vi "Recieve Status.vi"(8 "error in (no error)":errorcluster, 9 "Status offset":u64, 10 "Read config instead":bool, 11 "RP Communicator in":refnum<class "RP Communicator.lvclass">) -> (0 "error out":errorcluster, 1 "Status response":u32=1 format="0x%x (%d)", 3 "RP Communicator out":refnum<class "RP Communicator.lvclass">)   [LabVIEW 2016, in "RP Communicator.lvclass"]
uses:
  RP Communicator.lvclass
  RP Communicator.lvclass/RP Communicator.ctl
  Read Timeout.vi
  RP Read Status TCP.vi
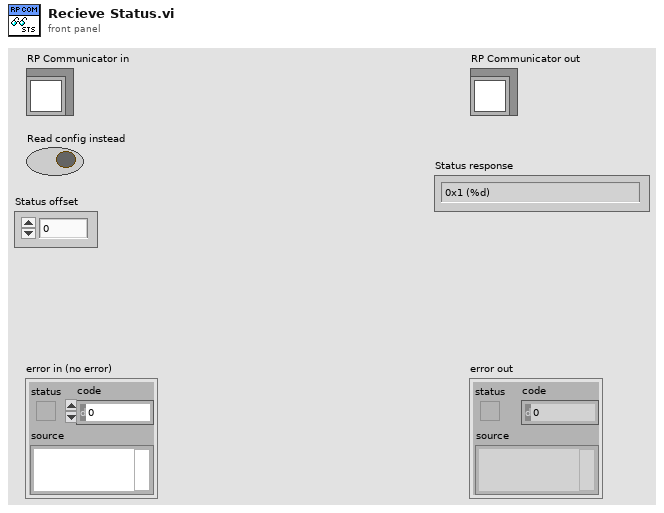
[diagram p1: front panel]
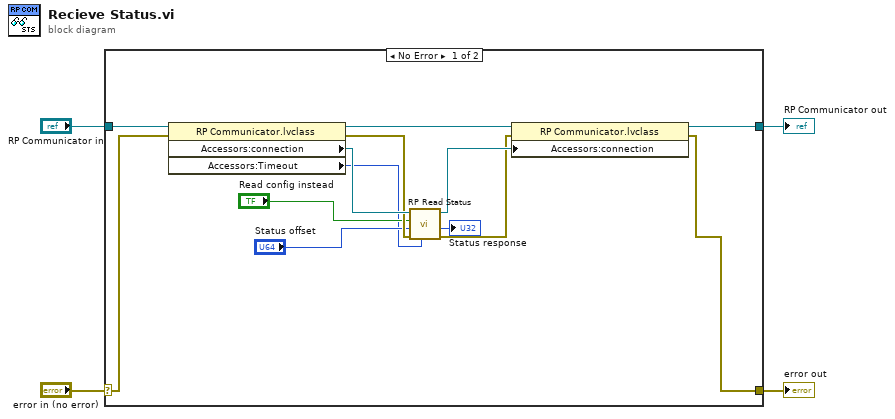
[diagram p0: block diagram]
diagram:
  n1 = case shown="No Error" "error in (no error)" {
    selector: "error in (no error)" -> [w9 w19]
    tunnel: [w11 w19] -> w3
    tunnel: [w14 w18] -> w1
    tunnel: "RP Communicator in" -> [w17 w18]
    frame No Error {
      n2 = property class="RP Communicator.lvclass"(reference=w17, error in=w9) -> (reference out=w16:refnum<class "RP Communicator.lvclass">, error out=w10:errorcluster, "Accessors:connection"=w15:refnum<k5>, "Accessors:Timeout"=w5:i32)
      n3 = call-poly "RP Read Status.vi"("timeout ms (25000)"=w5, "Error In"=w10, "Status offset"="Status offset", "Read config"="Read config instead", "connection ID"=w15) -> ("Error Out"=w12:errorcluster, "Status response"=→"Status response":u32, "connection ID out"=w13:refnum<k5>)  [unwired: 4 in]
      n4 = property class="RP Communicator.lvclass"(reference=w16, error in=w12, "Accessors:connection"=w13) -> (reference out=w14:refnum<class "RP Communicator.lvclass">, error out=w11:errorcluster)
    }
    frame Error {
    }
  }
  "error out" <- w3
  "RP Communicator out" <- w1
